vi "CAN Wrapper.vi"(6 "Signal Write":dbl, 7 "States":T1, 8 "error in":errorcluster, 9 "Setting":T2={"Termination"=1, "Baud Rate"=125000, "Interface"="CAN1", "XNET Database"="can_messages_818", "ECU"="GIP\ncan_messages_818"} {"Termination" items=["Off", "On"]}, 10 "Tx Signal In":string, 11 "Rx Signal In":string) -> (0 "error out":errorcluster={"status"=TRUE, "code"=-1074384711, "source"="XNET Create Session (Signal Input Single-point).vi:6590001<APPEND>\n\n<b>Complete call chain:</b>\r\n     XNET Create Session (Signal Input Single-point).vi:6590001\r\n     CAN GIP.lvlib:GIP CAN Wrapper.vi"}, 3 "Signal out":dbl=nan)   [LabVIEW 2021, in "CAN wrapper.lvlib"]
uses:
  CAN wrapper.lvlib
  Private Controls/Setting.ctl
  Private Controls/CAN States.ctl
  Private Controls/Local Variables.ctl
  <vilib>/JDP Science/JSONtext/Next JSON Value.vi
  <vilib>/JDP Science/JSONtext/String Subset.vi
  <vilib>/JDP Science/JSONtext/Parsing/Advance past next JSON Value (inlined COPY).vi
  <vilib>/JDP Science/JSONtext/Parsing/Advance past whitespace.vi
  <vilib>/JDP Science/JSONtext/Parsing/Advance past String.vi
  <vilib>/JDP Science/JSONtext/Parsing/Advance past Number.vi
  <vilib>/JDP Science/JSONtext/Parsing/Advance past Line Ending.vi
  <vilib>/xnet/xnet.llb/XNET Create Session (Signal Output Single-point).vi
  <vilib>/xnet/xnet.llb/XNET Create Session (Signal Input Single-point).vi
  <vilib>/xnet/xnet.llb/XNET Read (Signal Single-point).vi
  <vilib>/JDP Science/JSONtext/Parsing/Parse Full Path or Item Name.vi
  <vilib>/JDP Science/JSONtext/Parsing/Advance past Array.vi
  <vilib>/JDP Science/JSONtext/Parsing/Advance past Object.vi
  <vilib>/JDP Science/JSONtext/support/Error Cluster From Code.vi
  <vilib>/JDP Science/JSONtext/Offset/Find Item Locations by Path.vi
  <vilib>/xnet/xnet.llb/XNET Write (Signal Single-point).vi
  <resource>/objmgr/xnet.rc
  <vilib>/JDP Science/JSONtext/JSONtext.lvlib
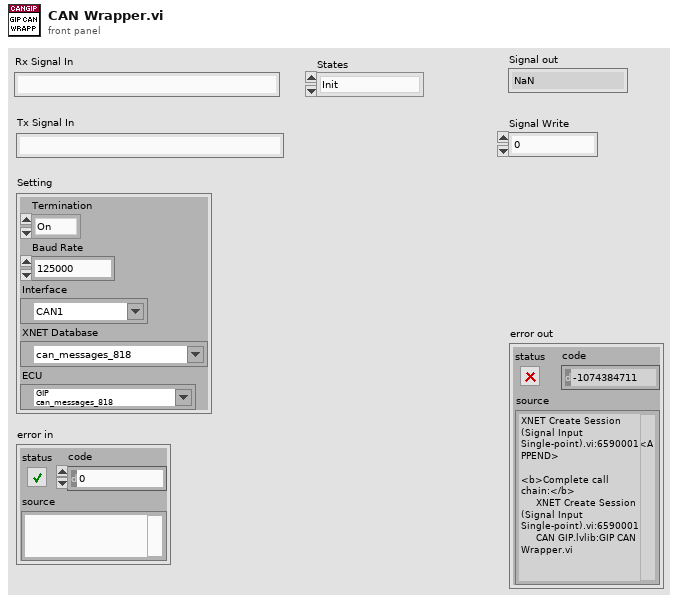
[diagram p1: front panel]
types:
  T1 = typedef "CAN wrapper.lvlib/CAN States.ctl" = enum16{"Init", "Config", "Read Signals", "Write Signals", "Close"}
  T2 = typedef "CAN wrapper.lvlib/Setting.ctl" = cluster{"Termination":u32, "Baud Rate":u64, "Interface":refnum<k21>, "XNET Database":refnum<k21>, "ECU":refnum<k21>}
  T3 = typedef "CAN wrapper.lvlib/Local Variables.ctl" = cluster{"Rx session":refnum<k21>, "Tx session":refnum<k21>, "Tx Data":dbl[], "JSON":string}
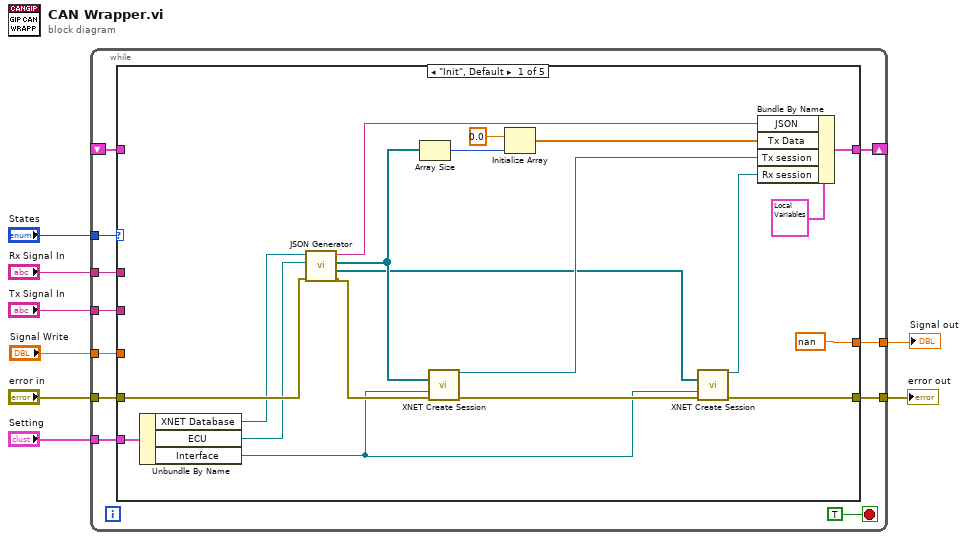
[diagram p0: block diagram]
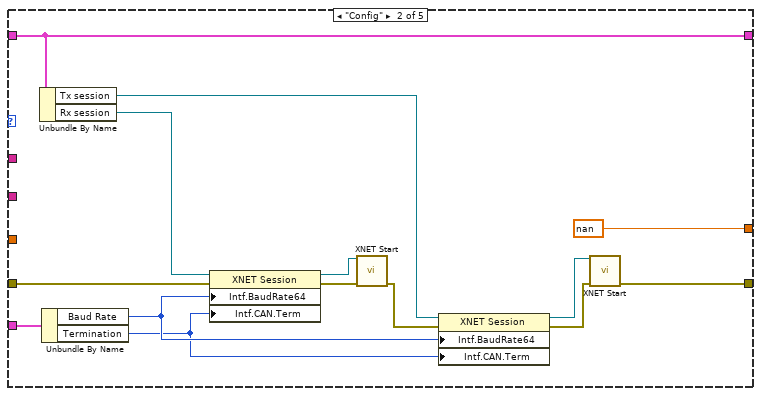
[diagram p2: hidden frame]
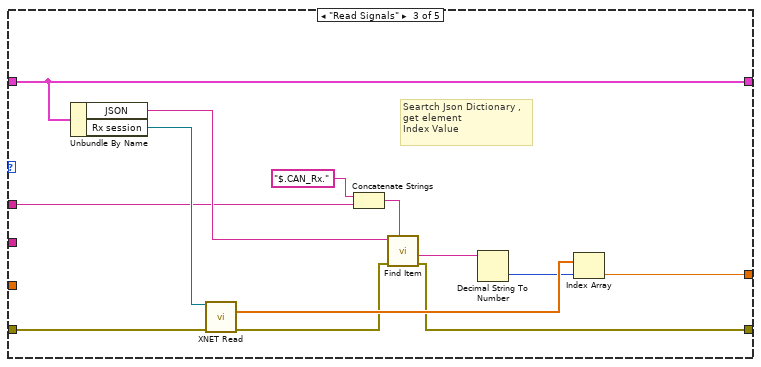
[diagram p3: hidden frame]
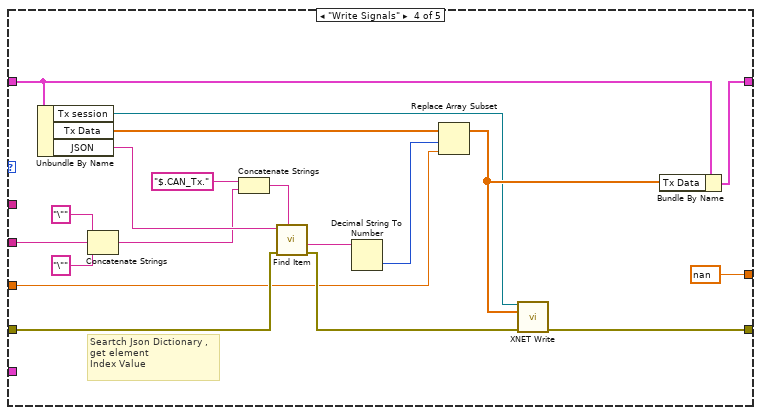
[diagram p4: hidden frame]
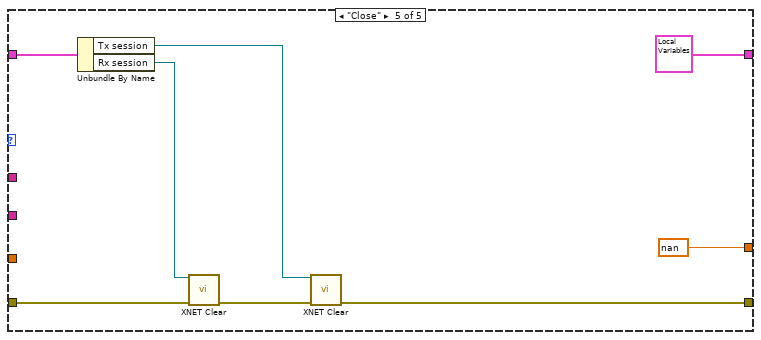
[diagram p5: hidden frame]
diagram:
  n1 = while {
    tunnel: "States" -> [w18]
    tunnel: "error in" -> [w17]
    tunnel: [w16] -> w7
    shift-right: [w15] -> _
    shift-left: _ -> [w14]
    tunnel: "Setting" -> [w13]
    tunnel: "Rx Signal In" -> [w12]
    tunnel: [w11] -> w3
    tunnel: "Signal Write" -> [w10]
    tunnel: "Tx Signal In" -> [w9]
    stop <- TRUE stop-if-true
    n2 = case shown="\"Init\", Default" w18 {
      tunnel: w17 -> [w32 w46 w65 w78 w92]
      tunnel: [w23 w42 w56 w66 w89] -> w16
      tunnel: [w37 w50 w63 w72 T3 {"Rx session"="", "Tx session"="", "Tx Data"=[], "JSON"="{\n  \"CAN_Rx\":{\n    \"GIP_GetPartNumber.lChar0\":0,\n    \"GIP_GetPartNumber.lChar1\":1,\n    \"GIP_GetPartNumber.lChar2\":2,\n    \"GIP_GetPartNumber.lChar3\":3,\n    \"GIP_GetPartNumber.lChar4\":4,\n    \"GIP_GetPartNumber.lChar5\":5,\n    \"GIP_GetPartNumber.lChar6\":6,\n    \"GIP_GetPartNumber.lChar7\":7,\n    \"GIP_GetPartNumber.rChar0\":8,\n    \"GIP_GetPartNumber.rChar1\":9,\n    \"GIP_GetSerialNumber.vendorChar0\":10,\n    \"GIP_GetSerialNumber.vendorChar1\":11,\n    \"GIP_GetSerialNumber.vendorChar2\":12,\n    \"GIP_GetSerialNumber.weekAndSerial\":13,\n    \"GIP_Grid_ActiveEnergyExported.GIP_Grid_ActiveEnergyExported_L1\":14,\n    \"GIP_Grid_ActiveEnergyExported.GIP_Grid_ActiveEnergyExported_L2\":15,\n    \"GIP_Grid_ActiveEnergyImported.GIP_Grid_ActiveEnergyImported_L1\":16,\n    \"GIP_Grid_ActiveEnergyImported.GIP_Grid_ActiveEnergyImported_L2\":17,\n    \"GIP_Grid_Power.GIP_Grid_ActivePower_L1\":18,\n    \"GIP_Grid_Power.GIP_Grid_ActivePower_L2\":19,\n    \"GIP_Grid_Power.GIP_Grid_ReactivePower_L1\":20,\n    \"GIP_Grid_Power.GIP_Grid_ReactivePower_L2\":21,\n    \"GIP_Grid_TotalActiveEnergy.GIP_Grid_TotalActiveEnergyExported\":22,\n    \"GIP_Grid_TotalActiveEnergy.GIP_Grid_TotalActiveEnergyImported\":23,\n    \"GIP_Load_ActiveEnergyExported.GIP_Load_ActiveEnergyExported_L1\":24,\n    \"GIP_Load_ActiveEnergyExported.GIP_Load_ActiveEnergyExported_L2\":25,\n    \"GIP_Load_ActiveEnergyImported.GIP_Load_ActiveEnergyImported_L1\":26,\n    \"GIP_Load_ActiveEnergyImported.GIP_Load_ActiveEnergyImported_L2\":27,\n    \"GIP_Load_Power.GIP_Load_ActivePower_L1\":28,\n    \"GIP_Load_Power.GIP_Load_ActivePower_L2\":29,\n    \"GIP_Load_Power.GIP_Load_ReactivePower_L1\":30,\n    \"GIP_Load_Power.GIP_Load_ReactivePower_L2\":31,\n    \"GIP_Load_TotalActiveEnergy.GIP_Load_TotalActiveEnergyExported\":32,\n    \"GIP_Load_TotalActiveEnergy.GIP_Load_TotalActiveEnergyImported\":33,\n    \"GIP_Status.GIP_Relay_State\":34,\n    \"GIP_Status.GIP_State\":35\n  },\n  \"CAN_Tx\":{\n    \"GIP_ManufacturingControl.ESP32Comms\":0,\n    \"GIP_ManufacturingControl.FaultLED\":1,\n    \"GIP_ManufacturingControl.Relay\":2,\n    \"GIP_ManufacturingControl.ST8500Comms\":3,\n    \"GIP_ManufacturingControl.StatusLED\":4,\n    \"GIP_SetPartNumber.lChar0\":5,\n    \"GIP_SetPartNumber.lChar1\":6,\n    \"GIP_SetPartNumber.lChar2\":7,\n    \"GIP_SetPartNumber.lChar3\":8,\n    \"GIP_SetPartNumber.lChar4\":9,\n    \"GIP_SetPartNumber.lChar5\":10,\n    \"GIP_SetPartNumber.lChar6\":11,\n    \"GIP_SetPartNumber.lChar7\":12,\n    \"GIP_SetPartNumber.rChar0\":13,\n    \"GIP_SetPartNumber.rChar1\":14,\n    \"GIP_SetSerialNumber.vendorChar0\":15,\n    \"GIP_SetSerialNumber.vendorChar1\":16,\n    \"GIP_SetSerialNumber.vendorChar2\":17,\n    \"GIP_SetSerialNumber.weekAndSerial\":18,\n    \"GIP_SetTestedFlag.GIP_TestedFlag\":19,\n    \"GIP_TestMode.GIP_TestModeFlag\":20\n  }\n}"}] -> w15
      tunnel: w14 -> [_ w50 w63 w75 w91]
      tunnel: w13 -> [w29 w51 _ _ _]
      tunnel: w12 -> [_ _ w54 _ _]
      tunnel: [nan nan w61 nan nan] -> w11
      tunnel: w10 -> [_ _ _ w76 _]
      tunnel: w9 -> [_ _ _ w70 _]
      frame "Init", Default {
        n3 = Unbundle By Name(w29) -> ("XNET Database"=w28:refnum<k21>, "ECU"=w27:refnum<k21>, "Interface"=w22:refnum<k21>)
        n4 = call "JSON Generator.vi"("error in (no error)"=w32, "ECU"=w27, "XNET Database"=w28) -> ("error out"=w25:errorcluster, "Rx Sigs"=w20:refnum<k21>[], "Tx Sigs"=w26:refnum<k21>[], "JSON"=w31:string)  [unwired: 5 in]
        n5 = Array Size(array=w26) -> (size(s)=w36:i32)
        n6 = call-poly <vilib>:"XNET Create Session.vi"("signal list"=w26, "interface"=w22, "error in (no error)"=w25) -> ("session out"=w30:refnum<k21>, "error out"=w24:errorcluster)  [unwired: 11 out]
        n7 = Initialize Array(0.0 ("element"), w36) -> (w34:dbl[])
        n8 = call-poly <vilib>:"XNET Create Session.vi"("signal list"=w20, "interface"=w22, "error in (no error)"=w24) -> ("session out"=w21:refnum<k21>, "error out"=w23:errorcluster)  [unwired: 11 out]
        n9 = Bundle By Name(cluster=T3 {"Rx session"="", "Tx session"="", "Tx Data"=[], "JSON"="{\n  \"CAN_Rx\":{\n    \"GIP_GetPartNumber.lChar0\":0,\n    \"GIP_GetPartNumber.lChar1\":1,\n    \"GIP_GetPartNumber.lChar2\":2,\n    \"GIP_GetPartNumber.lChar3\":3,\n    \"GIP_GetPartNumber.lChar4\":4,\n    \"GIP_GetPartNumber.lChar5\":5,\n    \"GIP_GetPartNumber.lChar6\":6,\n    \"GIP_GetPartNumber.lChar7\":7,\n    \"GIP_GetPartNumber.rChar0\":8,\n    \"GIP_GetPartNumber.rChar1\":9,\n    \"GIP_GetSerialNumber.vendorChar0\":10,\n    \"GIP_GetSerialNumber.vendorChar1\":11,\n    \"GIP_GetSerialNumber.vendorChar2\":12,\n    \"GIP_GetSerialNumber.weekAndSerial\":13,\n    \"GIP_Grid_ActiveEnergyExported.GIP_Grid_ActiveEnergyExported_L1\":14,\n    \"GIP_Grid_ActiveEnergyExported.GIP_Grid_ActiveEnergyExported_L2\":15,\n    \"GIP_Grid_ActiveEnergyImported.GIP_Grid_ActiveEnergyImported_L1\":16,\n    \"GIP_Grid_ActiveEnergyImported.GIP_Grid_ActiveEnergyImported_L2\":17,\n    \"GIP_Grid_Power.GIP_Grid_ActivePower_L1\":18,\n    \"GIP_Grid_Power.GIP_Grid_ActivePower_L2\":19,\n    \"GIP_Grid_Power.GIP_Grid_ReactivePower_L1\":20,\n    \"GIP_Grid_Power.GIP_Grid_ReactivePower_L2\":21,\n    \"GIP_Grid_TotalActiveEnergy.GIP_Grid_TotalActiveEnergyExported\":22,\n    \"GIP_Grid_TotalActiveEnergy.GIP_Grid_TotalActiveEnergyImported\":23,\n    \"GIP_Load_ActiveEnergyExported.GIP_Load_ActiveEnergyExported_L1\":24,\n    \"GIP_Load_ActiveEnergyExported.GIP_Load_ActiveEnergyExported_L2\":25,\n    \"GIP_Load_ActiveEnergyImported.GIP_Load_ActiveEnergyImported_L1\":26,\n    \"GIP_Load_ActiveEnergyImported.GIP_Load_ActiveEnergyImported_L2\":27,\n    \"GIP_Load_Power.GIP_Load_ActivePower_L1\":28,\n    \"GIP_Load_Power.GIP_Load_ActivePower_L2\":29,\n    \"GIP_Load_Power.GIP_Load_ReactivePower_L1\":30,\n    \"GIP_Load_Power.GIP_Load_ReactivePower_L2\":31,\n    \"GIP_Load_TotalActiveEnergy.GIP_Load_TotalActiveEnergyExported\":32,\n    \"GIP_Load_TotalActiveEnergy.GIP_Load_TotalActiveEnergyImported\":33,\n    \"GIP_Status.GIP_Relay_State\":34,\n    \"GIP_Status.GIP_State\":35\n  },\n  \"CAN_Tx\":{\n    \"GIP_ManufacturingControl.ESP32Comms\":0,\n    \"GIP_ManufacturingControl.FaultLED\":1,\n    \"GIP_ManufacturingControl.Relay\":2,\n    \"GIP_ManufacturingControl.ST8500Comms\":3,\n    \"GIP_ManufacturingControl.StatusLED\":4,\n    \"GIP_SetPartNumber.lChar0\":5,\n    \"GIP_SetPartNumber.lChar1\":6,\n    \"GIP_SetPartNumber.lChar2\":7,\n    \"GIP_SetPartNumber.lChar3\":8,\n    \"GIP_SetPartNumber.lChar4\":9,\n    \"GIP_SetPartNumber.lChar5\":10,\n    \"GIP_SetPartNumber.lChar6\":11,\n    \"GIP_SetPartNumber.lChar7\":12,\n    \"GIP_SetPartNumber.rChar0\":13,\n    \"GIP_SetPartNumber.rChar1\":14,\n    \"GIP_SetSerialNumber.vendorChar0\":15,\n    \"GIP_SetSerialNumber.vendorChar1\":16,\n    \"GIP_SetSerialNumber.vendorChar2\":17,\n    \"GIP_SetSerialNumber.weekAndSerial\":18,\n    \"GIP_SetTestedFlag.GIP_TestedFlag\":19,\n    \"GIP_TestMode.GIP_TestModeFlag\":20\n  }\n}"}, "JSON"=w31, "Tx Data"=w34, "Tx session"=w30, "Rx session"=w21) -> (w37:T3)
      }
      frame "Config" {
        n10 = Unbundle By Name(w50) -> ("Tx session"=w49:refnum<k21>, "Rx session"=w52:refnum<k21>)
        n11 = Unbundle By Name(w51) -> ("Baud Rate"=w48:u64, "Termination"=w47:u32)
        n12 = property class="XNET Session"(reference=w52, error in=w46, "Intf.BaudRate64"=w48, "Intf.CAN.Term"=w47) -> (reference out=w43:refnum<k21>, error out=w45:errorcluster)
        n13 = call <vilib>:"XNET Start.vi"("session in"=w43, "error in (no error)"=w45) -> ("error out"=w44:errorcluster)  [unwired: 12 in, 1 out]
        n14 = property class="XNET Session"(reference=w49, error in=w44, "Intf.BaudRate64"=w48, "Intf.CAN.Term"=w47) -> (reference out=w40:refnum<k21>, error out=w41:errorcluster)
        n15 = call <vilib>:"XNET Start.vi"("session in"=w40, "error in (no error)"=w41) -> ("error out"=w42:errorcluster)  [unwired: 12 in, 1 out]
      }
      frame "Read Signals" {
        # "Seartch Json Dictionary ,\nget element\nIndex Value"
        n16 = Unbundle By Name(w63) -> ("JSON"=w58:string, "Rx session"=w64:refnum<k21>)
        n17 = call-poly <vilib>:"XNET Read.vi"("session in"=w64, "error in (no error)"=w65) -> ("data"=w62:dbl[], "error out"=w57:errorcluster)  [unwired: 12 out]
        n18 = Concatenate Strings("$.CAN_Rx." ("$Path or Item Name"), w54) -> (w59:string)
        n19 = call <vilib>:"Find Item.vi"("$Path or Item Name"=w59, "error in (no error)"=w57, "JSON"=w58) -> ("error out"=w56:errorcluster, "<JSON>"=w53:string)  [unwired: 5 in, 2 out]
        n20 = Decimal String To Number(string=w53) -> (number=w55:i32)  [unwired: 2 in, 1 out]
        n21 = Index Array(array=w62, index=w55) -> (element=w61:dbl)
      }
      frame "Write Signals" {
        # "Seartch Json Dictionary ,\nget element\nIndex Value"
        n22 = Unbundle By Name(w75) -> ("Tx session"=w71:refnum<k21>, "Tx Data"=w74:dbl[], "JSON"=w80:string)
        n23 = Concatenate Strings("\"" ("string"), w70, "\"" ("string")) -> (w68:string)
        n24 = Concatenate Strings("$.CAN_Tx." ("$Path or Item Name"), w68) -> (w81:string)
        n25 = call <vilib>:"Find Item.vi"("$Path or Item Name"=w81, "error in (no error)"=w78, "JSON"=w80) -> ("error out"=w77:errorcluster, "<JSON>"=w83:string)  [unwired: 5 in, 2 out]
        n26 = Decimal String To Number(string=w83) -> (number=w79:i32)  [unwired: 2 in, 1 out]
        n27 = Replace Array Subset(array=w74, new element=w76, index=w79) -> (w73:dbl[])
        n28 = call-poly <vilib>:"XNET Write.vi"("session in"=w71, "data"=w73, "error in (no error)"=w77) -> ("error out"=w66:errorcluster)  [unwired: 12 out]
        n29 = Bundle By Name(cluster=w75, "Tx Data"=w73) -> (w72:T3)
      }
      frame "Close" {
        n30 = Unbundle By Name(w91) -> ("Tx session"=w87:refnum<k21>, "Rx session"=w88:refnum<k21>)
        n31 = call <vilib>:"XNET Clear.vi"("session in"=w88, "error in (no error)"=w92) -> ("error out"=w90:errorcluster)  [unwired: 13 in]
        n32 = call <vilib>:"XNET Clear.vi"("session in"=w87, "error in (no error)"=w90) -> ("error out"=w89:errorcluster)  [unwired: 13 in]
      }
    }
  }
  "error out" <- w7
  "Signal out" <- w3
